vi "Resize.Resize X-Y Graph within Tab Ctrl.vi"(5 "Pix from Bottom":i32, 6 "Min Size":cluster{"Width":i32, "Height":i32}={"Width"=250, "Height"=200}, 7 "Pix from Right":i32, 8 "error in":errorcluster, 9 "Aspect Ratio":cluster{"W/H":dbl, "Enable":bool}={"W/H"=1.0, "Enable"=FALSE} {"W/H" format="%.2g"}, 10 "X-Y Graph Ctrl":refnum<vi>, 11 "Tab Ctrl":refnum<vi>) -> (0 "error out":errorcluster, 2 "X-Y Graph Ctrl Out":refnum<vi>, 3 "Tab Ctrl Out":refnum<vi>)   [LabVIEW 2024, in "EQMF.lvlib" / "Controls.lvlib"]
uses:
  Controls.lvlib
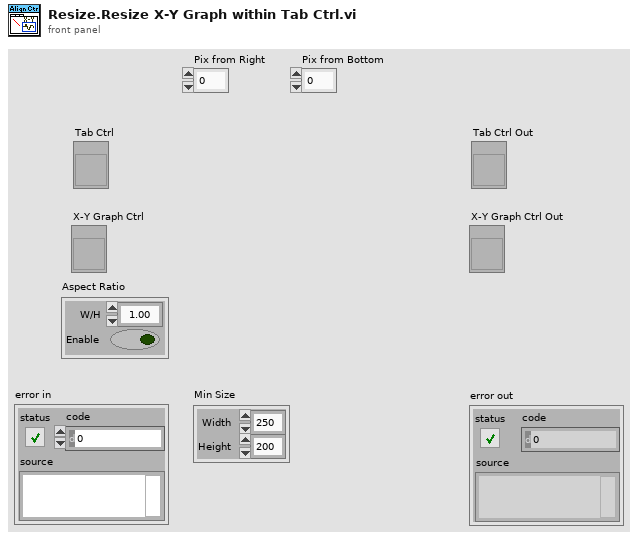
[diagram p1: front panel]
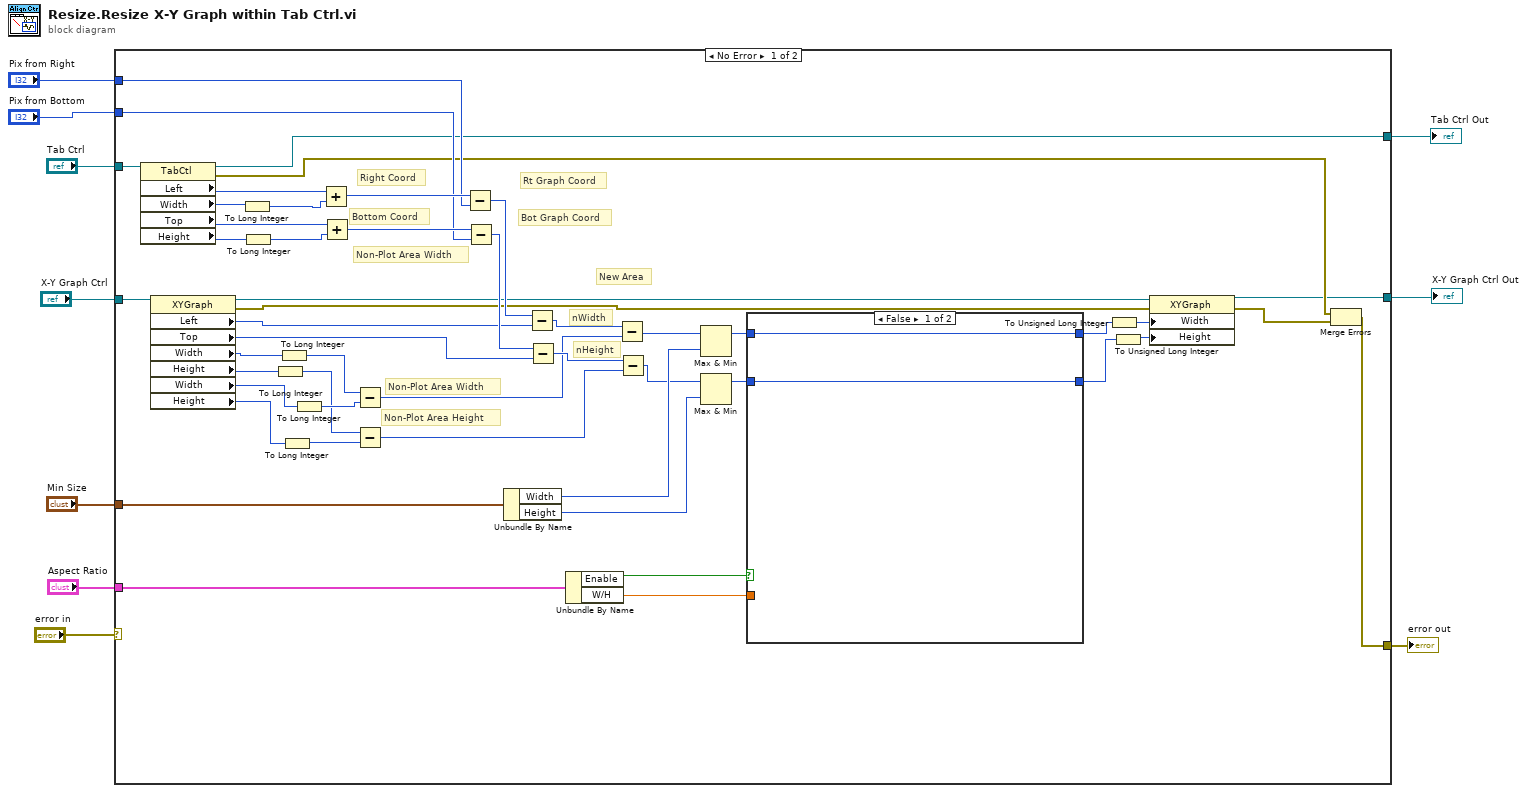
[diagram p0: block diagram]
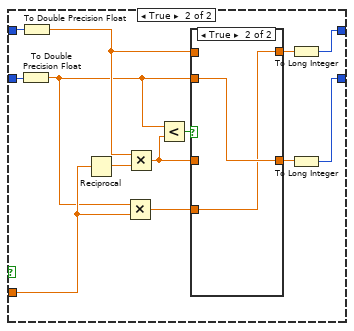
[diagram p2: hidden frame]
diagram:
  n1 = case shown="No Error" "error in" {
    selector: "error in" -> [_ w79]
    tunnel: "Pix from Right" -> [w43 _]
    tunnel: "Pix from Bottom" -> [w42 _]
    tunnel: [w31 w79] -> w8
    tunnel: "Min Size" -> [w30 _]
    tunnel: "Aspect Ratio" -> [w23 _]
    tunnel: "Tab Ctrl" -> [w20 w81]
    tunnel: "X-Y Graph Ctrl" -> [w19 w80]
    tunnel: [w16 w81] -> w3
    tunnel: [w15 w80] -> w2
    frame No Error {
      # "nHeight"
      # "nWidth"
      # "New Area"
      # "Bot Graph Coord"
      # "Rt Graph Coord"
      # "Non-Plot Area Width"
      # "Bottom Coord"
      # "Right Coord"
      # "Non-Plot Area Height"
      # "Non-Plot Area Width"
      n2 = property on="Property Node" class="TabCtl"(reference=w20) -> (reference out=w16:refnum<vi>, error out=w18:errorcluster, "Left"=w47:i32, "Width"=w50:u32, "Top"=w48:i32, "Height"=w49:u32)  [unwired: 1 in]
      n3 = property on="Property Node" class="XYGraph"(reference=w19) -> (reference out=w33:refnum<vi>, error out=w32:errorcluster, "Left"=w39:i32, "Top"=w38:i32, "Width"=w46:u32, "Height"=w59:u32, "Width"=w58:u32, "Height"=w57:u32)  [unwired: 1 in]
      n4 = To Long Integer(number=w50) -> (32bit integer=w51:i32)
      n5 = To Long Integer(number=w49) -> (32bit integer=w52:i32)
      n6 = To Long Integer(number=w59) -> (32bit integer=w54:i32)
      n7 = To Long Integer(number=w46) -> (32bit integer=w55:i32)
      n8 = To Long Integer(number=w57) -> (32bit integer=w53:i32)
      n9 = To Long Integer(number=w58) -> (32bit integer=w56:i32)
      n10 = Add(x=w47, y=w51) -> (x+y=w44:i32)
      n11 = Add(x=w48, y=w52) -> (x+y=w45:i32)
      n12 = Subtract(x=w55, y=w56) -> (x-y=w35:i32)
      n13 = Subtract(x=w54, y=w53) -> (x-y=w34:i32)
      n14 = Subtract(x=w44, y=w43) -> (x-y=w41:i32)
      n15 = Subtract(x=w45, y=w42) -> (x-y=w40:i32)
      n16 = Unbundle By Name(w30) -> ("Width"=w29:i32, "Height"=w28:i32)
      n17 = Subtract(x=w41, y=w39) -> (x-y=w37:i32)
      n18 = Subtract(x=w40, y=w38) -> (x-y=w36:i32)
      n19 = Unbundle By Name(w23) -> ("Enable"=w22:bool, "W/H"=w21:dbl)
      n20 = Subtract(x=w37, y=w35) -> (x-y=w26:i32)
      n21 = Subtract(x=w36, y=w34) -> (x-y=w27:i32)
      n22 = Max & Min(x=w26, y=w29) -> (max(x,y)=w25:i32)  [unwired: 1 out]
      n23 = Max & Min(x=w27, y=w28) -> (max(x,y)=w24:i32)  [unwired: 1 out]
      n24 = case shown="False" w22 {
        tunnel: w25 -> [w61 w74]
        tunnel: w24 -> [w60 w73]
        tunnel: [w61 w65] -> w11
        tunnel: [w60 w66] -> w12
        tunnel: w21 -> [_ w71]
        frame False {
        }
        frame True {
          n25 = To Double Precision Float(number=w73) -> (double precision float=w63:dbl)
          n26 = To Double Precision Float(number=w74) -> (double precision float=w70:dbl)
          n27 = Reciprocal(x=w71) -> (1/x=w72:dbl)
          n28 = Multiply(x=w63, y=w71) -> (x*y=w62:dbl)
          n29 = Multiply(x=w70, y=w72) -> (x*y=w69:dbl)
          n30 = Less?(x=w63, y=w69) -> (x < y?=w68:bool)
          n31 = case shown="True" w68 {
            tunnel: w70 -> [w76 _]
            tunnel: w69 -> [w75 _]
            tunnel: [w76 w77] -> w64
            tunnel: [w75 w78] -> w67
            tunnel: w63 -> [_ w78]
            tunnel: w62 -> [_ w77]
            frame False {
            }
            frame True {
            }
          }
          n32 = To Long Integer(number=w64) -> (32bit integer=w65:i32)
          n33 = To Long Integer(number=w67) -> (32bit integer=w66:i32)
        }
      }
      n34 = To Unsigned Long Integer(number=w11) -> (unsigned 32bit integer=w14:u32)
      n35 = To Unsigned Long Integer(number=w12) -> (unsigned 32bit integer=w13:u32)
      n36 = property on="Property Node" class="XYGraph"(reference=w33, error in=w32, "Width"=w14, "Height"=w13) -> (reference out=w15:refnum<vi>, error out=w17:errorcluster)
      n37 = Merge Errors(w18, w17) -> (w31:errorcluster)
    }
    frame Error {
    }
  }
  "error out" <- w8
  "Tab Ctrl Out" <- w3
  "X-Y Graph Ctrl Out" <- w2
